vi "Read.vi"(8 "error in (no error)":errorcluster, 9 "Starting independent variable":dbl, 10 "Current independent variable":dbl, 11 "PC Reader in":refnum<class "PC Reader.lvclass">) -> (0 "error out":errorcluster, 2 "Data Channels":T1, 3 "PC Reader out":refnum<class "PC Reader.lvclass">)   [LabVIEW 2009, in "PC Reader.lvclass"]
doc: "Prepare for read, wait the time delay, and take data from up to 4 channels."
uses:
  PC Reader.lvclass
  Instruments/Utility Classes/Readable/Data Channels.ctl
  Instruments/Utility Classes/Readable/Data Channel.ctl
  Instruments/Utility Classes/Readable/Data Point.ctl
  PC Reader.lvclass/PC Reader.ctl
  Instruments/Utility Classes/Readable/Readable.lvclass
  Reader/Reader.lvclass
  Instruments/Photon Counter/SR400/SR400.lvlib
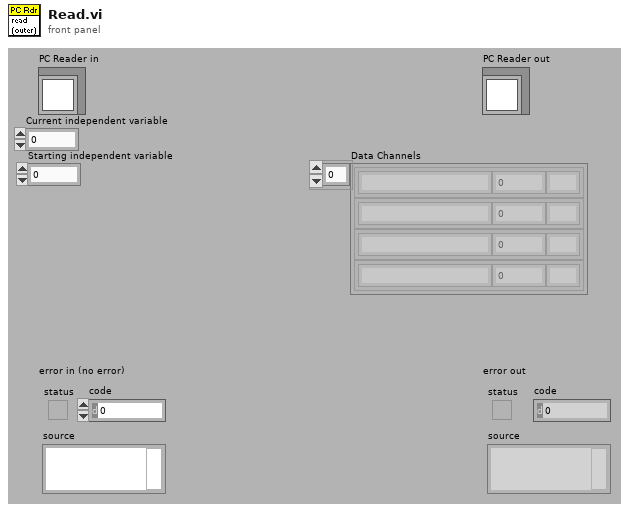
[diagram p1: front panel]
types:
  T1 = typedef "Readable.lvclass/Data Channels.ctl" = T2[]
  T2 = typedef "Readable.lvclass/Data Channel.ctl" = cluster{"Name":string, "Data Point":T3, "Unit":string}
  T3 = typedef "Readable.lvclass/Data Point.ctl" = dbl
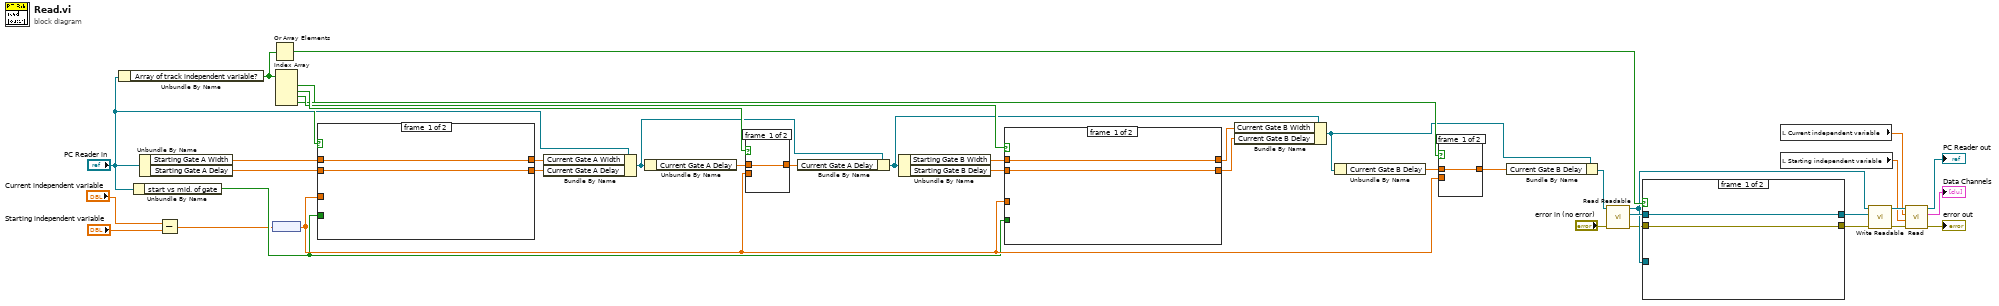
[diagram p0: block diagram]
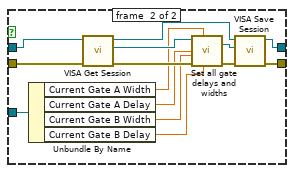
[diagram p2: hidden frame]
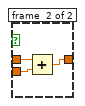
[diagram p3: hidden frame]
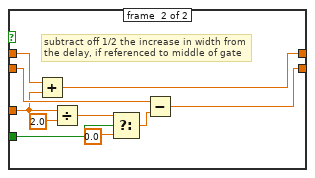
[diagram p4: hidden frame]
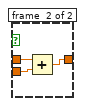
[diagram p5: hidden frame]
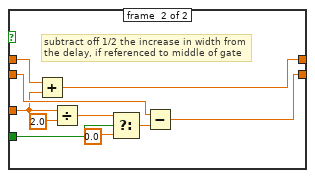
[diagram p6: hidden frame]
diagram:
  n1 = Unbundle By Name("PC Reader in") -> ("Array of track independent variable?"=w8:bool[])
  n2 = Unbundle By Name("PC Reader in") -> ("start vs mid. of gate"=w13:bool)
  n3 = Unbundle By Name("PC Reader in") -> ("Starting Gate A Width"=w38:dbl[unit], "Starting Gate A Delay"=w17:dbl[unit])
  n4 = Subtract(x="Current independent variable", y="Starting independent variable") -> (x-y=w9:dbl)
  n5 = node(w9) -> (w25:dbl[unit])
  n6 = Or Array Elements(Boolean array=w8) -> (logical OR=w7:bool)
  n7 = Index Array(array=w8) -> (element #1=w26:bool, element #2=w41:bool, element #3=w40:bool, element #4=w39:bool)  [unwired: 4 in]
  n8 = case shown="True" w26 {
    tunnel: w25 -> [_ w44]
    tunnel: w38 -> [w43 w53]
    tunnel: [w43 w47] -> w18
    tunnel: w13 -> [_ w51]
    tunnel: w17 -> [w42 w49]
    tunnel: [w42 w45] -> w16
    frame #0 {
    }
    frame #1 {
      # "subtract off 1/2 the increase in width from \nthe delay, if referenced to middle of gate"
      n9 = Add(x=w53, y=w44) -> (x+y=w47:dbl[unit])
      n10 = Divide(x=w44, y=2.0) -> (x/y=w46:dbl[unit])
      n11 = Select(t=w46, s=w51, f=dbl[unit] 0.0) -> (s? t:f=w52:dbl[unit])
      n12 = Subtract(x=w49, y=w52) -> (x-y=w45:dbl[unit])
    }
  }
  n13 = Bundle By Name(cluster="PC Reader in", "Current Gate A Width"=w18, "Current Gate A Delay"=w16) -> (w21:refnum<class "PC Reader.lvclass">)
  n14 = Unbundle By Name(w21) -> ("Current Gate A Delay"=w27:dbl[unit])
  n15 = case shown="True" w41 {
    tunnel: w25 -> [_ w56]
    tunnel: w27 -> [w54 w55]
    tunnel: [w54 w57] -> w24
    frame #0 {
    }
    frame #1 {
      n16 = Add(x=w55, y=w56) -> (x+y=w57:dbl[unit])
    }
  }
  n17 = Bundle By Name(cluster=w21, "Current Gate A Delay"=w24) -> (w20:refnum<class "PC Reader.lvclass">)
  n18 = Unbundle By Name(w20) -> ("Starting Gate B Width"=w28:dbl[unit], "Starting Gate B Delay"=w14:dbl[unit])
  n19 = case shown="True" w40 {
    tunnel: w25 -> [_ w60]
    tunnel: w28 -> [w59 w69]
    tunnel: [w59 w62] -> w23
    tunnel: [w58 w65] -> w15
    tunnel: w14 -> [w58 w64]
    tunnel: w13 -> [_ w63]
    frame #0 {
    }
    frame #1 {
      # "subtract off 1/2 the increase in width from \nthe delay, if referenced to middle of gate"
      n20 = Add(x=w69, y=w60) -> (x+y=w62:dbl[unit])
      n21 = Divide(x=w60, y=2.0) -> (x/y=w61:dbl[unit])
      n22 = Select(t=w61, s=w63, f=dbl[unit] 0.0) -> (s? t:f=w66:dbl[unit])
      n23 = Subtract(x=w64, y=w66) -> (x-y=w65:dbl[unit])
    }
  }
  n24 = Bundle By Name(cluster=w20, "Current Gate B Width"=w23, "Current Gate B Delay"=w15) -> (w19:refnum<class "PC Reader.lvclass">)
  n25 = Unbundle By Name(w19) -> ("Current Gate B Delay"=w29:dbl[unit])
  n26 = case shown="True" w39 {
    tunnel: w25 -> [_ w71]
    tunnel: w29 -> [w70 w72]
    tunnel: [w70 w73] -> w22
    frame #0 {
    }
    frame #1 {
      n27 = Add(x=w72, y=w71) -> (x+y=w73:dbl[unit])
    }
  }
  n28 = Bundle By Name(cluster=w19, "Current Gate B Delay"=w22) -> (w3:refnum<class "PC Reader.lvclass">)
  n29 = call-dynamic "Read Readable.vi"("error in (no error)"="error in (no error)", "Reader.lvclass in"=w3) -> ("error out"=w1:errorcluster, "Readable.lvclass"=w12:refnum<class "Readable.lvclass">, "Reader.lvclass out"=w4:refnum<class "PC Reader.lvclass">)  [unwired: 7 out]
  n30 = case shown="True" w7 {
    tunnel: w12 -> [w75 w89]
    tunnel: [w75 w88] -> w11
    tunnel: w1 -> [w74 w86]
    tunnel: [w74 w85] -> w10
    tunnel: w4 -> [_ w84]
    frame #0 {
    }
    frame #1 {
      n31 = Unbundle By Name(w84) -> ("Current Gate A Width"=w79:dbl[unit], "Current Gate A Delay"=w78:dbl[unit], "Current Gate B Width"=w77:dbl[unit], "Current Gate B Delay"=w76:dbl[unit])
      n32 = call-dynamic "VISA Get Session.vi"("error in (no error)"=w86, "Instrument.lvclass in"=w89) -> ("error out"=w81:errorcluster, "VISA Resource Name"=w83:refnum<visa-resource-name>, "Instrument.lvclass out"=w87:refnum<class "Readable.lvclass">)  [unwired: 7 out]
      n33 = call "Set all gate delays and widths.vi"("Gate B Delay (def: 0 s)"=w76, "Gate A Width (def: 0 s)"=w79, "error in (no error)"=w81, "Gate B Width (def: 0 s)"=w77, "Gate A Delay (def: 0 s)"=w78, "VISA resource name"=w83) -> ("error out"=w80:errorcluster, "VISA resource name out"=w82:refnum<visa-resource-name>)  [unwired: 4 out]
      n34 = call-dynamic "VISA Save Session.vi"("error in (no error)"=w80, "VISA Resource Name"=w82, "Instrument.lvclass in"=w87) -> ("error out"=w85:errorcluster, "Instrument.lvclass out"=w88:refnum<class "Readable.lvclass">)  [unwired: 7 out]
    }
  }
  n35 = local read "Current independent variable"() -> (w31:dbl)
  n36 = local read "Starting independent variable"() -> (w30:dbl)
  n37 = call-dynamic "Write Readable.vi"("error in (no error)"=w10, "Readable.lvclass"=w11, "Reader.lvclass in"=w4) -> ("error out"=w35:errorcluster, "Reader.lvclass out"=w33:refnum<class "PC Reader.lvclass">)  [unwired: 7 out]
  n38 = call-parent "Read.vi"("error in (no error)"=w35, "Starting independent variable"=w30, "Current independent variable"=w31, "Reader in"=w33) -> ("error out"=→"error out":errorcluster, "Data Channels"=→"Data Channels":T1, "Reader out"=→"PC Reader out":refnum<class "PC Reader.lvclass">)  [unwired: 5 out]
